vi "CLFNFixup.vi"   [LabVIEW 2020]
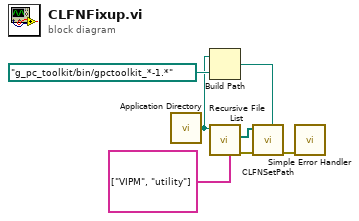
[diagram p0: block diagram]
diagram:
  n1 = call <vilib>:"Application Directory.vi"() -> ("Application Directory"=w1:path)
  n2 = Build Path(base path=w1, name or relative path=path "g_pc_toolkit/bin/gpctoolkit_*-1.*" ("New Path")) -> (appended path=w2:path)
  n3 = call <vilib>:"Recursive File List.vi"("Folders to Exclude"=string[] ["VIPM", "utility"], "Folder Path"=w1) -> ("error out"=w4:errorcluster, "All Files in Dir"=w6:path[])  [unwired: 5 in, 3 out]
  n4 = call "CLFNSetPath.vi"("New Path"=w2, "error in (no error)"=w4, "Files"=w6) -> ("error out"=w5:errorcluster)  [unwired: 7 in, 1 out]
  n5 = call <vilib>:"Simple Error Handler.vi"("error in (no error)"=w5) -> ()  [unwired: 4 in, 5 out]
